vi "GEECS tcp open single variable.vi"(8 "error in (no error)":errorcluster, 10 "Variable name":string, 11 "Device name":string) -> (0 "error out":errorcluster, 2 "String":string, 3 "TCP Network Connection out":refnum<k5>)   [LabVIEW 2020]
uses:
  MySQL/Preset Query Enum.ctl
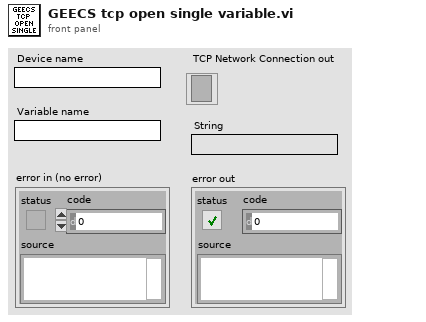
[diagram p1: front panel]
types:
  T1 = typedef "Preset Query Enum.ctl" = enum16{"Get Locations", "Get all IPs and MACs", "Get classes", "Get expt variables to set at scanstart for particular device", "Get expt devices and variables with start values", "Get expt devices and variables (with data to get)", "Get expt devices with data to get", "Get Expt devices and GUIs", "Get all devices basic properties", "Get Virtual Devices Core Info", "Get Expt names", "Get experiment basic properties", "Get experiment alarm variables", "Get MC Ports", "Get device network comm port", "Get devicetype lvclass path", "Get basic device properties", "Get Init Order", "Get all setable variables of a device", "Get device variable aliases", "Get force values of all settable variables", "Get all variables of a devicetype", "Get all variables of a device", "Get plotter details", "Get Saved Scans", "Get Scan Info", "GetGeneralGUIs", "Get expt for plotter", "Get plotter IDs from expt", "Get all devices", "Get all Virtual Devices", "Get all aliases", "Get variable and device info for Virtual Device", "GetItemLocatorIP", "Get IPs for GUIs", "Get DeviceType from Device", "GetLocalPortRange", "GetDevicePresetVariables", "Get Device Configuration", "GetAllPresetNames", "GetAllConfigurationNames", "GetPresetDeviceNames", "GetDeviceAliases", "GetDevicesOfClass"}
  T2 = typedef "UDP send cluster.ctl" = cluster{"IP Address":string, "UDP Port":string, "Command to Send":string}
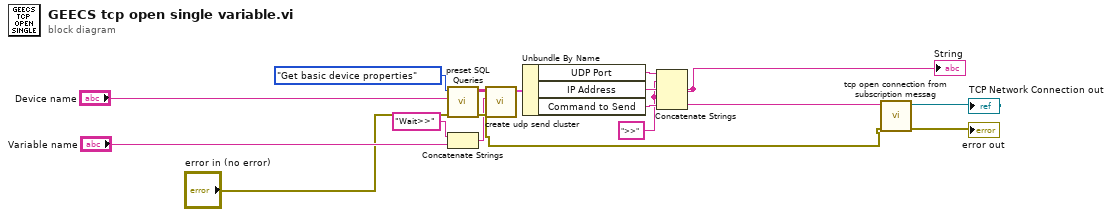
[diagram p0: block diagram]
diagram:
  w6 = ">>" ("string")
  n1 = call "preset SQL Queries.vi"("error in (no error)"="error in (no error)", "Device/Devicetype name\n/Plotter.id/ScanName#"="Device name", "Preset Query"=Preset_Query_Enum."Get basic device properties") -> ("error out"=w15:errorcluster, "data"=w3:string[][])  [unwired: 6 in, 1 out]
  n2 = Concatenate Strings("Wait>>" ("Remaining States"), "Variable name") -> (w12:string)
  n3 = call "create udp send cluster.vi"("Command to send"=w12, "Device Basic Properties"=w3) -> ("UDP Send Cluster"=w5:T2)  [unwired: 9 in]
  n4 = Unbundle By Name(w5) -> ("UDP Port"=w9:string, "IP Address"=w10:string, "Command to Send"=w11:string)
  n5 = Concatenate Strings(w9, w6, w10, w6, w11) -> (w13:string)
  "String" <- w13
  n6 = call "tcp open connection from subscription messag.vi"("error in (no error)"=w15, "subscribe message for process vi"=w13) -> ("error out"=→"error out":errorcluster, "TCP Network Connection out"=→"TCP Network Connection out":refnum<k5>)  [unwired: 8 in]
